vi "Send Trigger.vi"(8 "error in (no error)":errorcluster, 11 "SimELoad in":refnum<class "SimEload.lvclass">) -> (0 "error out":errorcluster, 2 "Trigger Time":timestamp, 3 "SimELoad out":refnum<class "SimEload.lvclass">)   [LabVIEW 2019, in "SimELoad.lvlib" / "SimEload.lvclass"]
uses:
  SimEload.lvclass
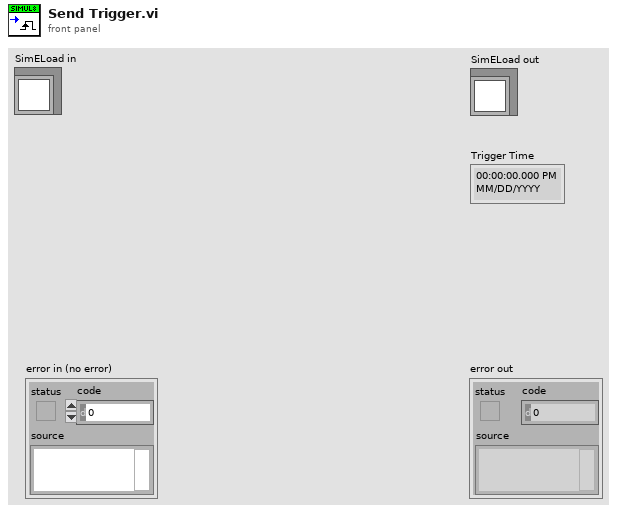
[diagram p1: front panel]
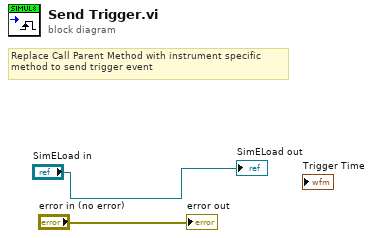
[diagram p0: block diagram]
diagram:
  # "Replace Call Parent Method with instrument specific\nmethod to send trigger event"
  "error out" <- "error in (no error)"
  "SimELoad out" <- "SimELoad in"
